vi "Set Error Handler.vi"(8 "error in (no error)":errorcluster, 10 "Error Handler":refnum<class "Error Handler Interface.lvclass">, 11 "Process In":refnum<class "Process.lvclass">) -> (0 "error out":errorcluster, 3 "Process Out":refnum<class "Process.lvclass">)   [LabVIEW 2020, in "Process.lvclass"]
doc: "Set the error handler for the process. The error handler Handle Errors.vi interface is then called by the Handle Process Errors.vi method."
uses:
  Process.lvclass
  Error Handler Interface/Error Handler Interface.lvclass
  Process.lvclass/Process.ctl
  <vilib>/AdvancedString/1D String Array to Delimited String.vi
  <vilib>/Utility/error.llb/Error Cluster From Error Code.vi
  <vilib>/ErrorRing/Error Ring.xnode
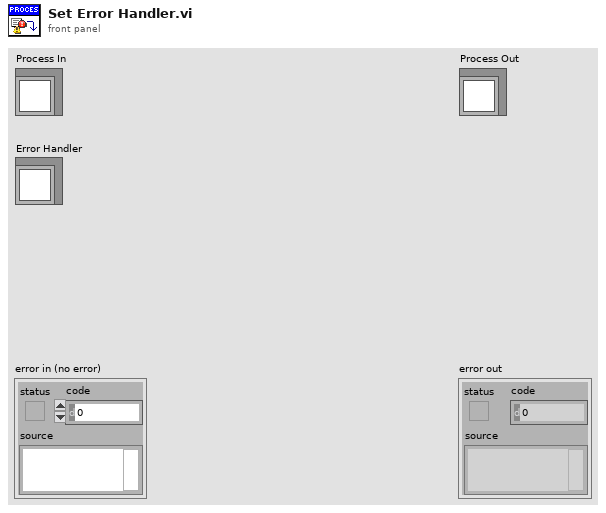
[diagram p1: front panel]
types:
  T1 = typedef "Process.lvclass/Lifecycle State.ctl" = enum16{"Uninitialized", "Initialized", "Started", "Running", "Stopped", "Finished"}
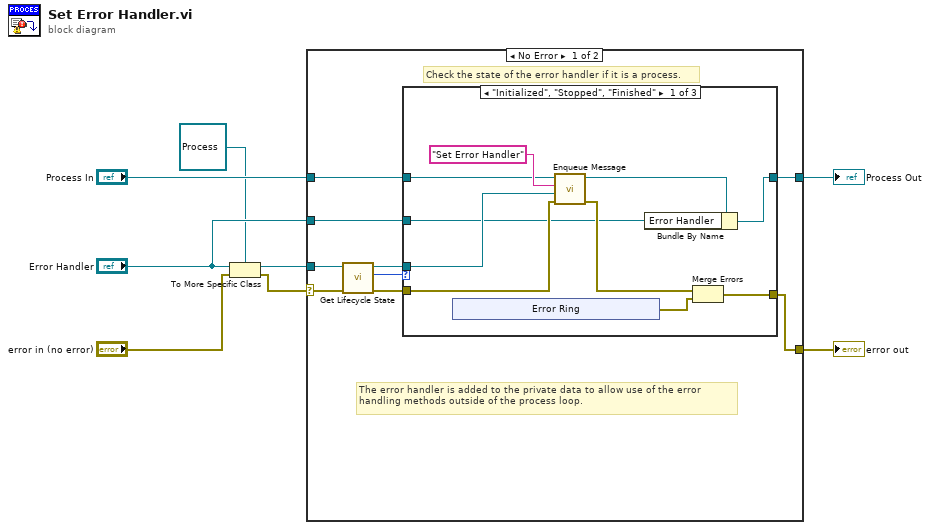
[diagram p0: block diagram]
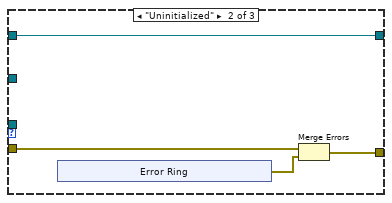
[diagram p2: hidden frame]
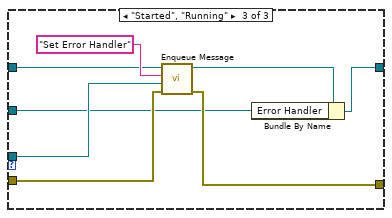
[diagram p3: hidden frame]
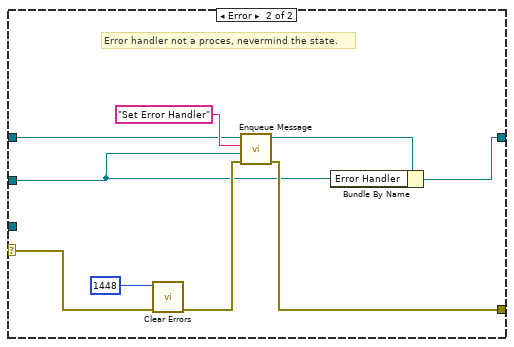
[diagram p4: hidden frame]
diagram:
  n1 = To More Specific Class(target class=refnum<class "Process.lvclass"> refnum ("Process.lvclass"), reference="Error Handler", error in="error in (no error)") -> (specific class reference=w3:refnum<class "Process.lvclass">, error out=w1:errorcluster)
  n2 = case shown="No Error" w1 {
    selector: w1 -> [w16 w56]
    tunnel: [w13 w49] -> w8
    tunnel: [w11 w51] -> w7
    tunnel: "Process In" -> [w12 w52]
    tunnel: w3 -> [w17 _]
    tunnel: "Error Handler" -> [w9 w48]
    frame No Error {
      # "The error handler is added to the private data to allow use of the error handling methods outside of the process loop."
      # "Check the state of the error handler if it is a process."
      n3 = call "Get Lifecycle State.vi"("error in (no error)"=w16, "Process In"=w17) -> ("error out"=w14:errorcluster, "Lifecycle State"=w15:T1, "Process Out"=w10:refnum<class "Process.lvclass">)  [unwired: 6 in, 1 out]
      n4 = case shown="\"Initialized\", \"Stopped\", \"Finished\"" w15 {
        tunnel: [w27 w35 w44] -> w13
        tunnel: w14 -> [w21 w33 w45]
        tunnel: w12 -> [w23 w32 w46]
        tunnel: [w19 w32 w42] -> w11
        tunnel: w10 -> [w22 _ w41]
        tunnel: w9 -> [w18 _ w40]
        frame "Initialized", "Stopped", "Finished" {
          n5 = xnode "Error Ring"() -> ("error out"=w26:errorcluster)
          n6 = call "Enqueue Message.vi"("error in (no error)"=w21, "Message Data"=w22, "Message"="Set Error Handler", "Process In"=w23) -> ("error out"=w20:errorcluster, "Process Out"=w24:refnum<class "Process.lvclass">)  [unwired: 6 in]
          n7 = Bundle By Name(cluster=w24, "Error Handler"=w18) -> (w19:refnum<class "Process.lvclass">)
          n8 = Merge Errors(w20, w26) -> (w27:errorcluster)
        }
        frame "Uninitialized" {
          n9 = xnode "Error Ring"() -> ("error out"=w34:errorcluster)
          n10 = Merge Errors(w33, w34) -> (w35:errorcluster)
        }
        frame "Started", "Running" {
          n11 = call "Enqueue Message.vi"("error in (no error)"=w45, "Message Data"=w41, "Message"="Set Error Handler", "Process In"=w46) -> ("error out"=w44:errorcluster, "Process Out"=w43:refnum<class "Process.lvclass">)  [unwired: 6 in]
          n12 = Bundle By Name(cluster=w43, "Error Handler"=w40) -> (w42:refnum<class "Process.lvclass">)
        }
      }
    }
    frame Error {
      # "Error handler not a proces, nevermind the state."
      n13 = call <vilib>:"Clear Errors.vi"("error in (no error)"=w56, "specific error code to clear (0: all)"=1448) -> ("error out"=w50:errorcluster)  [unwired: 4 in, 1 out]
      n14 = call "Enqueue Message.vi"("error in (no error)"=w50, "Message Data"=w48, "Message"="Set Error Handler", "Process In"=w52) -> ("error out"=w49:errorcluster, "Process Out"=w54:refnum<class "Process.lvclass">)  [unwired: 6 in]
      n15 = Bundle By Name(cluster=w54, "Error Handler"=w48) -> (w51:refnum<class "Process.lvclass">)
    }
  }
  "error out" <- w8
  "Process Out" <- w7
